vi "hse-configuration_GetAllKeysForSection.vi"(8 "error in (no error)":errorcluster, 10 "Section":string, 11 "hse-config-ini in":refnum<class "hse-config-ini.lvclass">) -> (0 "error out":errorcluster, 2 "Keys":string[](array[string]), 3 "hse-config-ini out":refnum<class "hse-config-ini.lvclass">)   [LabVIEW 2014, in "hse-config-ini.lvclass"]
doc: "Reads the numeric configuration value (DOUBLE) identified by <b>section</b> and <b>key</b> from the configuration object\n\n____\nHAMPEL SOFTWARE ENGINEERING v0.12.0 (2018-09-13 18:21)"
uses:
  hse-config-ini.lvclass
  hse-configuration.lvclass/hse-configuration.ctl
  hse-configuration_ReadDataDirectory.vi
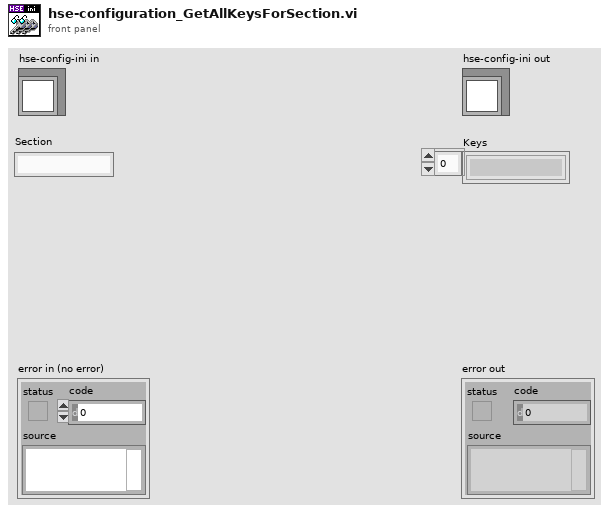
[diagram p1: front panel]
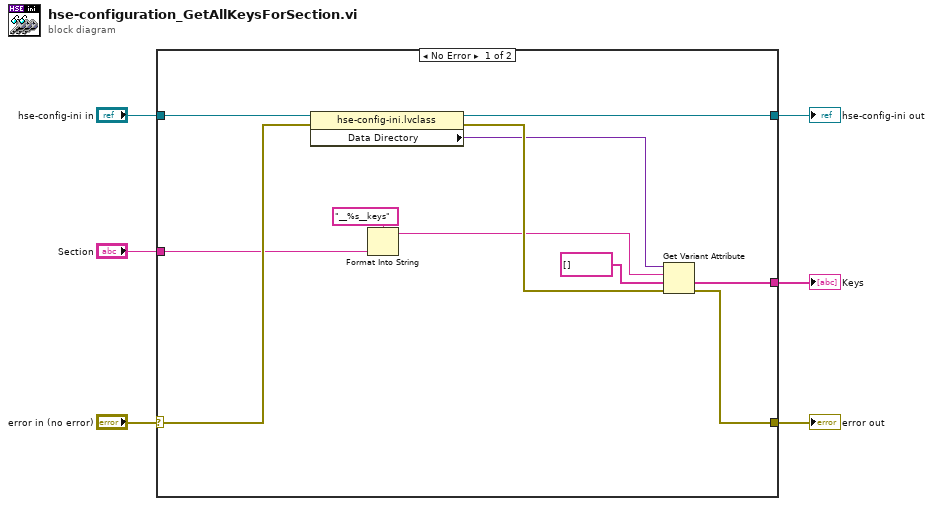
[diagram p0: block diagram]
diagram:
  n1 = case shown="No Error" "error in (no error)" {
    selector: "error in (no error)" -> [w15 w19]
    tunnel: [w13 w19] -> w3
    tunnel: "hse-config-ini in" -> [w17 w18]
    tunnel: [w16 w18] -> w4
    tunnel: [w10 _] -> w2
    tunnel: "Section" -> [w7 _]
    frame No Error {
      n2 = property class="hse-config-ini.lvclass"(reference=w17, error in=w15) -> (reference out=w16:refnum<class "hse-config-ini.lvclass">, error out=w14:errorcluster, "Data Directory"=w12:variant)
      n3 = Format Into String(format string="__%s__keys" ("name"), w7) -> (resulting string=w8:string)  [unwired: 2 in, 1 out]
      n4 = Get Variant Attribute(Variant=w12, name=w8, default value (empty Variant)=string[] [] ("Sections"), error in=w14) -> (value=w10:string[], error out=w13:errorcluster)  [unwired: 2 out]
    }
    frame Error {
    }
  }
  "error out" <- w3
  "hse-config-ini out" <- w4
  "Keys" <- w2
